vi "面积与周长.vi"(11 "测量结果":cluster{"Area":dbl, "Perimeter":dbl} {"Perimeter" format="%.2f"; "Area" format="%.2f"}) -> (2 "周长":dbl, 3 "面积":dbl)   [LabVIEW 2015]
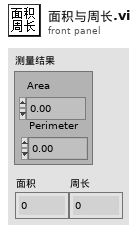
[diagram p1: front panel]
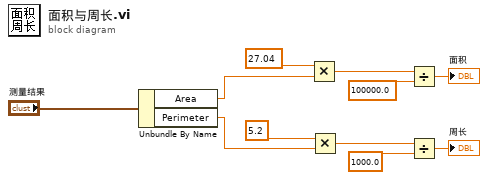
[diagram p0: block diagram]
diagram:
  n1 = Unbundle By Name("测量结果") -> ("Area"=w11:dbl, "Perimeter"=w9:dbl)
  n2 = Multiply(x=27.04, y=w11) -> (x*y=w7:dbl)
  n3 = Multiply(x=5.2, y=w9) -> (x*y=w5:dbl)
  n4 = Divide(x=w7, y=100000.0) -> (x/y=→"面积":dbl)
  n5 = Divide(x=w5, y=1000.0) -> (x/y=→"周长":dbl)
